vi "Main-Temp.vi"   [LabVIEW 2019]
uses:
  <vilib>/ActorFramework/Actor/Actor.lvclass
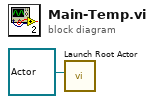
[diagram p0: block diagram]
diagram:
  n1 = call <vilib>:"Launch Root Actor.vi"("Actor"=refnum<class "Actor.lvclass"> refnum) -> ()  [unwired: 9 in, 2 out]
